vi "Clear errors from TWM.vi"(8 "error in (no error)":errorcluster, 10 "pipe name":string="\\\\.\\pipe\\TWM:server", 11 "handle in":i32) -> (0 "open error out":errorcluster, 3 "handle out":i32, 4 "original error out":errorcluster)   [LabVIEW 2020]
doc: "Clears errors from TWM pipe by closing pipe connection and opening again. This VI changes pipe reference! Temporary replacement until TWM library will fix impossibility to clear errors from the TWM server."
uses:
  external libraries/TWM-1.8.7.0-client/TWM Client.lvlib
  external libraries/varilib/varilib.lvlib
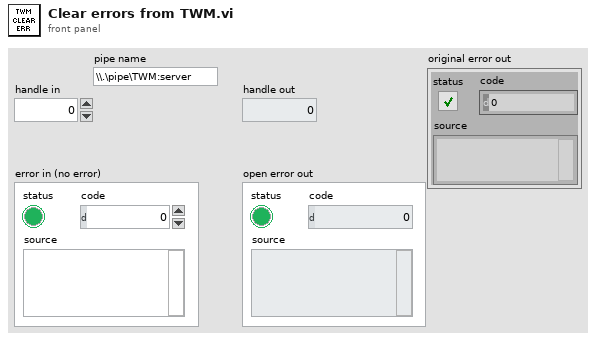
[diagram p1: front panel]
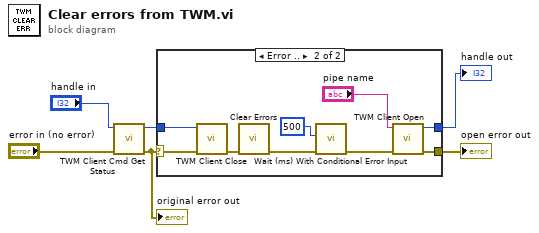
[diagram p0: block diagram]
diagram:
  n1 = call "TWM Client Cmd Get Status.vi"("error in"="error in (no error)", "handle"="handle in") -> ("error out"=w5:errorcluster, "handle out"=w1:i32)  [unwired: 5 in, 3 out]
  "original error out" <- w5
  n2 = case shown="Error .." w5 {
    selector: w5 -> [w7 w12]
    tunnel: [w7 w11] -> w4
    tunnel: [w8 w10] -> w3
    tunnel: w1 -> [w8 w9]
    frame No Error {
    }
    frame Error {
      n3 = call "TWM Client Close.vi"("error in"=w12, "handle in"=w9) -> ("error out"=w14:errorcluster)  [unwired: 9 in]
      n4 = call <vilib>:"Clear Errors.vi"("error in (no error)"=w14) -> ("error out"=w15:errorcluster)  [unwired: 5 in, 1 out]
      n5 = call "Wait (ms) With Conditional Error Input.vi"("error in (no error)"=w15, "milliseconds to wait"=u32 500) -> ("error out"=w16:errorcluster)  [unwired: 8 in, 1 out]
      n6 = call "TWM Client Open.vi"("error in"=w16, "pipe name"="pipe name") -> ("error out"=w11:errorcluster, "handle out"=w10:i32)  [unwired: 8 in]
    }
  }
  "open error out" <- w4
  "handle out" <- w3
